vi "OpenProj.vi"(3 "entrée d'erreur":errorcluster) -> (0 "sortie d'erreur":errorcluster, 2 "NomProjet":string)   [LabVIEW 2017]
panel:
  in  "Ouvrir":bool
  in  "Projets":i32(listbox)=1
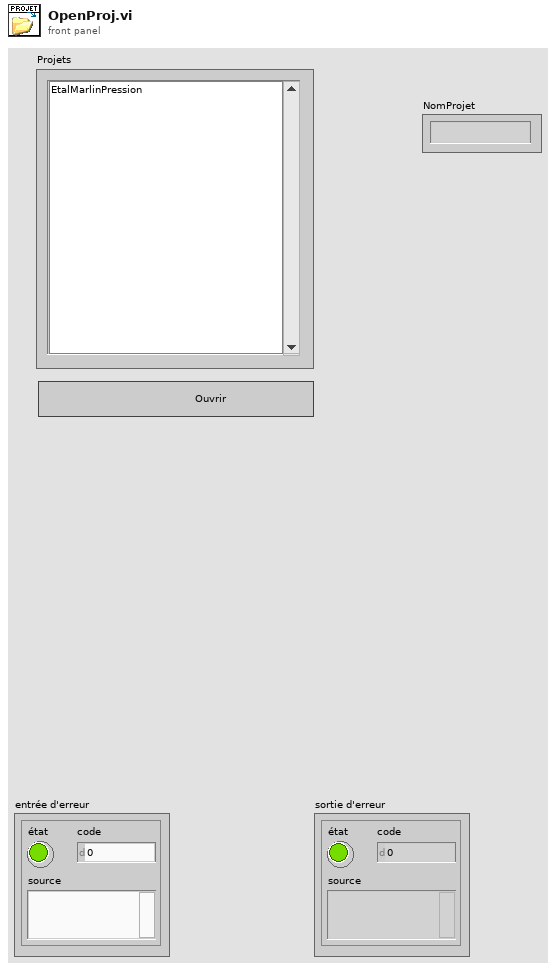
[diagram p1: front panel]
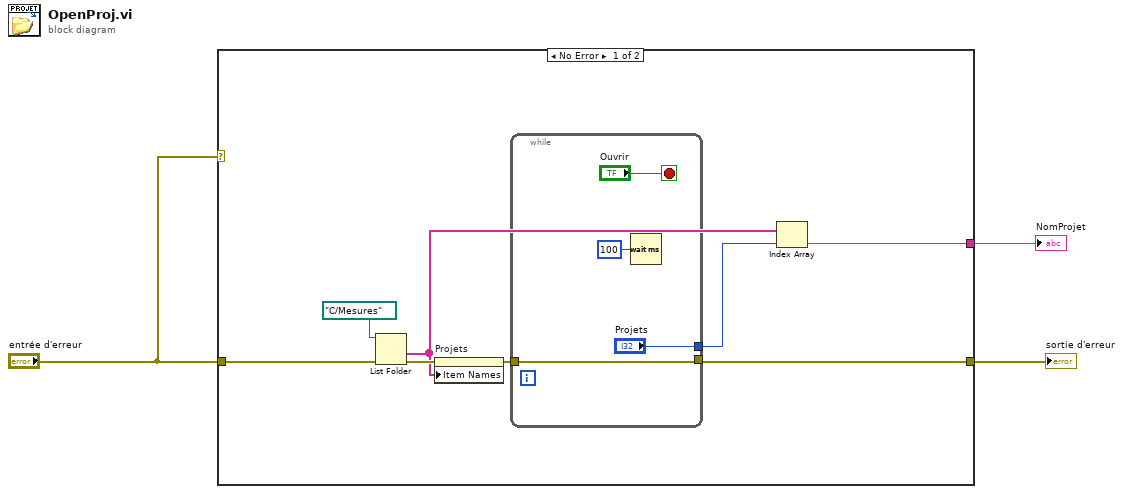
[diagram p0: block diagram]
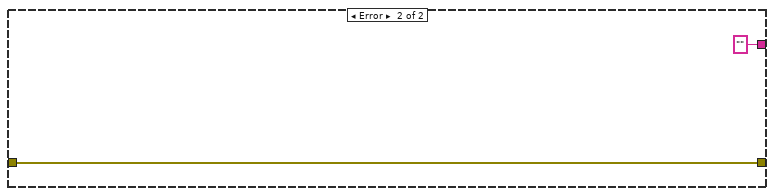
[diagram p2: hidden frame]
diagram:
  n1 = case shown="No Error" "entrée d'erreur" {
    tunnel: [w5 w17] -> w3
    tunnel: "entrée d'erreur" -> [w11 w17]
    tunnel: [w4 ""] -> w1
    frame No Error {
      n2 = List Folder(path=path "C:/Mesures" ("chemin"), error in=w11) -> (folder names=w7:string[], error out=w9:errorcluster)  [unwired: 2 in, 2 out]
      n3 = property on="Projets" class="LstBox (strict)"(error in=w9, "Item Names"=w7) -> (error out=w8:errorcluster)  [unwired: 1 in, 1 out]
      n4 = while {
        tunnel: w8 -> [w14]
        tunnel: [w14] -> w5
        tunnel: ["Projets"] -> w6
        stop <- "Ouvrir" stop-if-true
        n5 = Wait (ms)(milliseconds to wait=u32 100 ("attente (ms)")) -> ()  [unwired: 1 out]
      }
      n6 = Index Array(array=w7, index=w6) -> (element=w4:string)
    }
    frame Error {
    }
  }
  "sortie d'erreur" <- w3
  "NomProjet" <- w1
